vi "TDK-Lambda GEN LAN Series - GUI Demo.vi"() -> ()   [LabVIEW 2025]
doc: "This is a simple Graphical User Interface (GUI), for the TDK-Lambda Genesys DC Power Supplies using Ethernet (LAN) ports. \n\nIt has controls and indicators that automatically update in an endless polling loop. It also shows a pop-up form when errors are detected.\n\nControls: \n- Knobs to set voltage and current limits.\n- Buttons to set the output on or off, reset and quit.\n\nIndicators:\n- Shows the measured output voltage and current.\n- Shows the CV or CC regulation mode.\n- Shows when the output is turned off.\n- Shows fault shut down messages."
uses:
  <userlib>/TDK-Lambda GEN LAN Series/TDK-Lambda GEN LAN Series.lvlib
panel:
  in  "Revision":string="Rev 1.03"
  in  "RESET":bool
  out "Seqnc":string
  in  "VISA Name":refnum<visa-resource-name>="TCPIP0::0.0.0.0::inst0::INSTR" caption="IP Address"
  out "Irate Str":string caption="I Rate"
  out "Vrate Str":string caption="V Rate"
  out "Console":string
  in  "PC":dbl(knob) min=0.0 max=25.0 scale=0.0..25.0 scale format="%.1f"
  in  "IDecPt":enum16{"1", "10", "100", "1000"}(ring)=enum."100"
  in  "VDecPt":enum16{"1", "10", "100", "1000"}(ring)=enum."100"
  in  "QuitBtn":bool
  out "CcLed":bool=TRUE
  out "OUTled":bool=TRUE
  in  "OUT":bool
  out "IDisp":cluster{string[], bool, bool, bool, bool}={["0", "0", "0", "0", "0"], FALSE, FALSE, TRUE, FALSE}
  out "CvLed":bool=TRUE
  out "VDisp":cluster{string[], bool, bool, bool, bool}={["0", "0", "0", "0", "0"], FALSE, TRUE, FALSE, FALSE}
  in  "PV":dbl(knob) min=0.0 max=30.0 scale=0.0..30.0 scale format="%.1f"
  # "Command Logging"
  # "GENESYS Power Supply"
  # "DC VOLTS"
  # "DC AMPS"
  # "(c) 2019 TDK-Lambda.  ALL RIGHTS RESERVED."
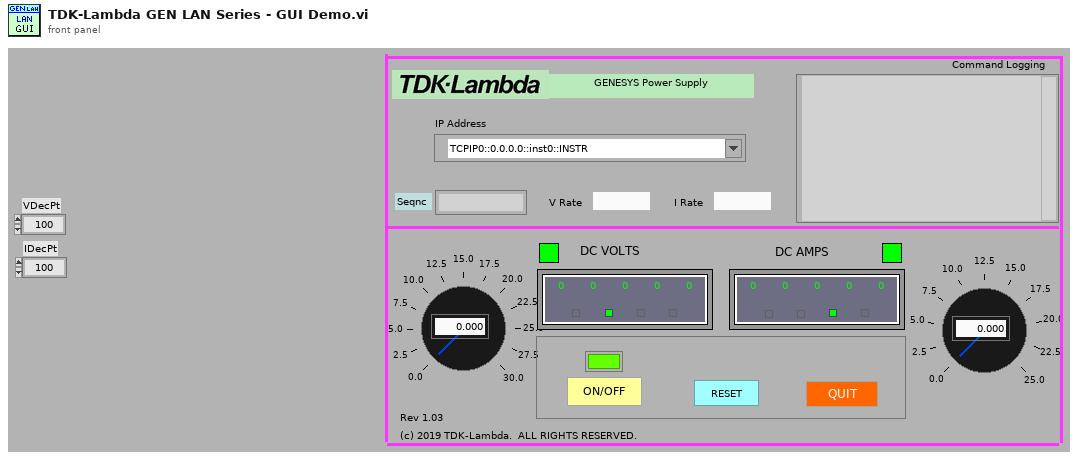
[diagram p1: front panel]
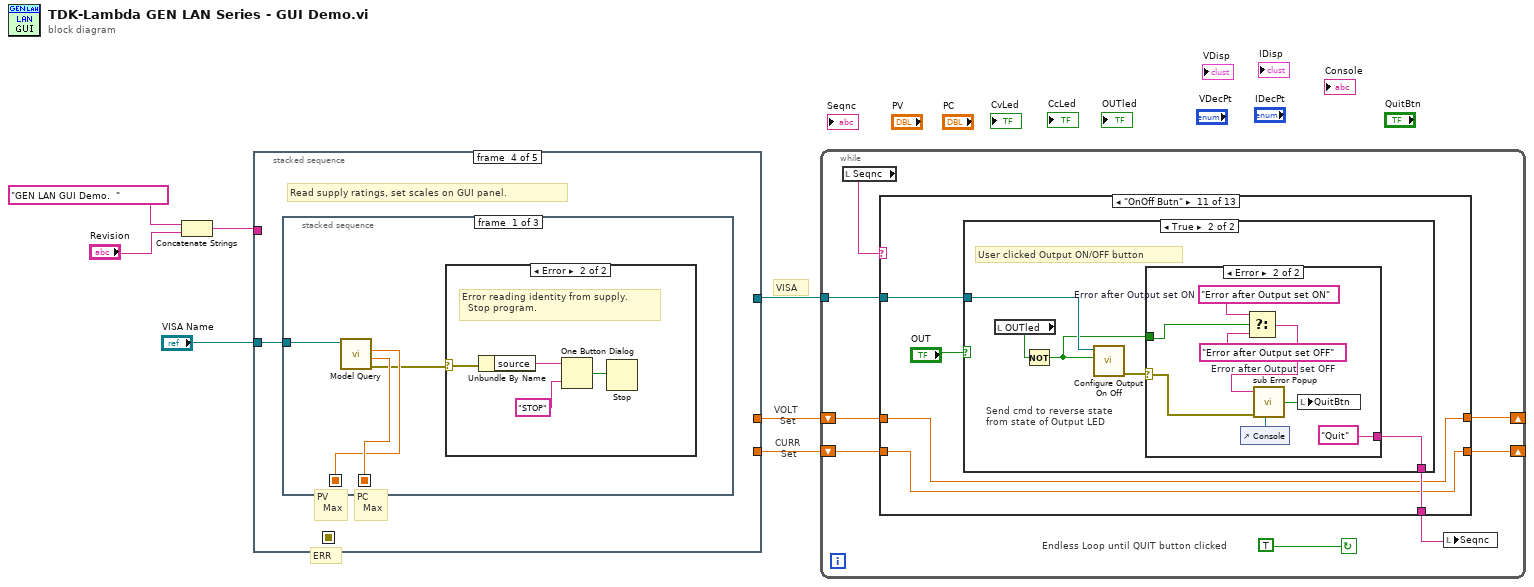
[diagram p0: block diagram]
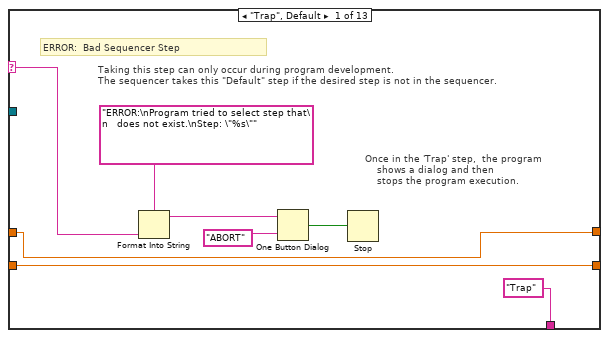
[diagram p2: hidden frame]
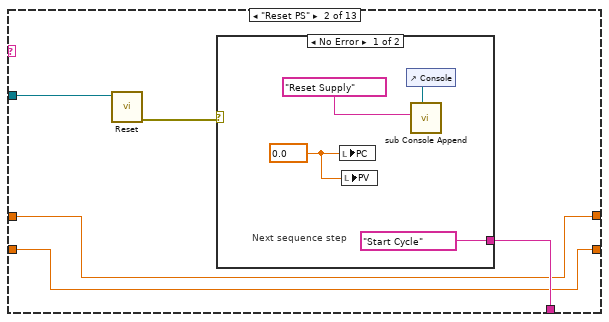
[diagram p3: hidden frame]
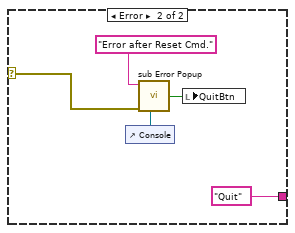
[diagram p4: hidden frame]
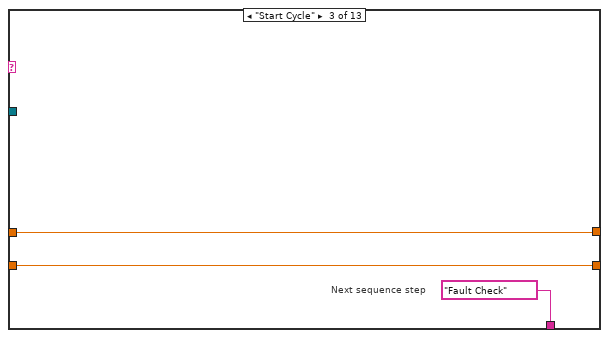
[diagram p5: hidden frame]
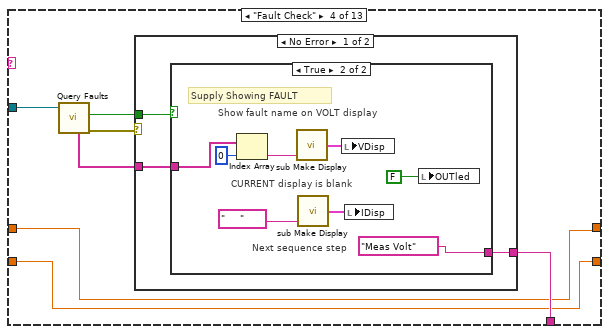
[diagram p6: hidden frame]
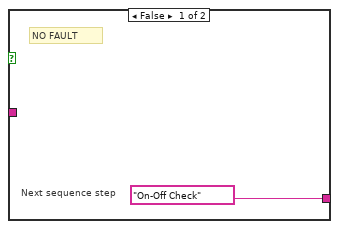
[diagram p7: hidden frame]
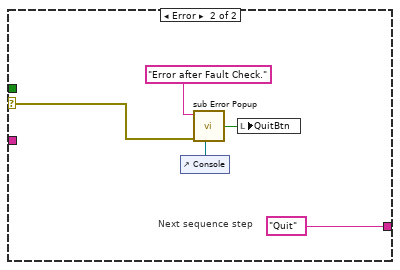
[diagram p8: hidden frame]
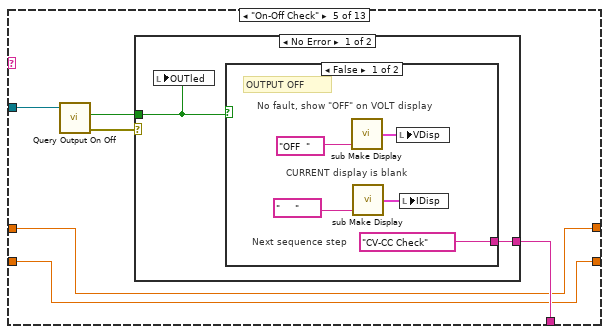
[diagram p9: hidden frame]
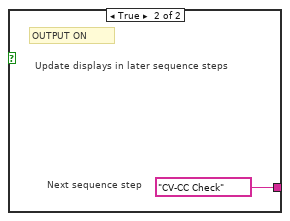
[diagram p10: hidden frame]
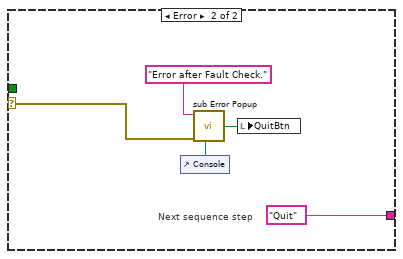
[diagram p11: hidden frame]
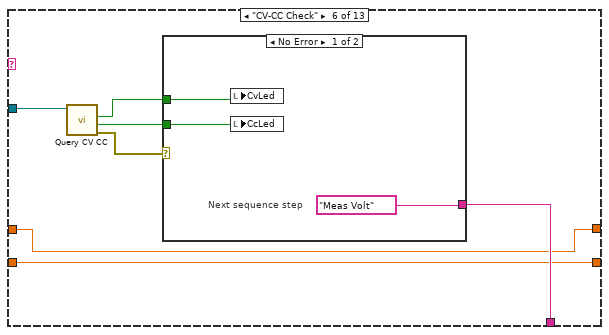
[diagram p12: hidden frame]
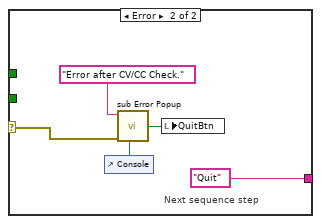
[diagram p13: hidden frame]
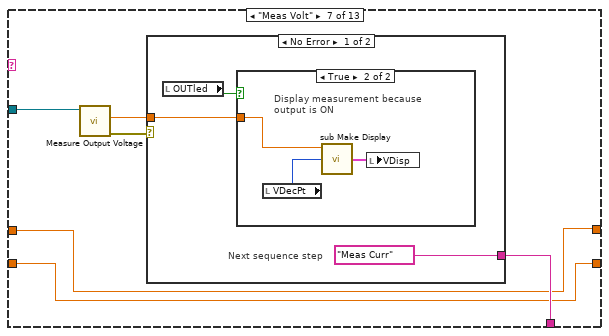
[diagram p14: hidden frame]
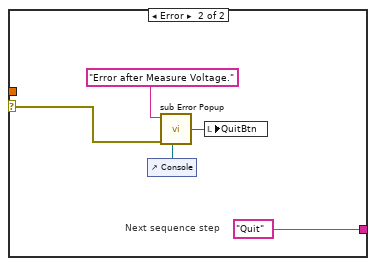
[diagram p16: hidden frame]
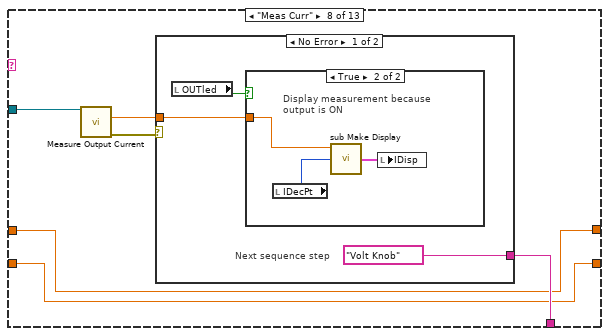
[diagram p17: hidden frame]
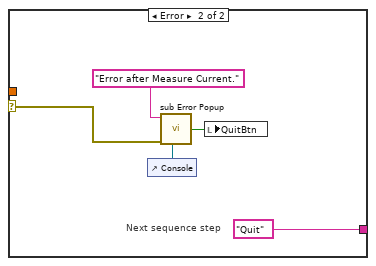
[diagram p19: hidden frame]
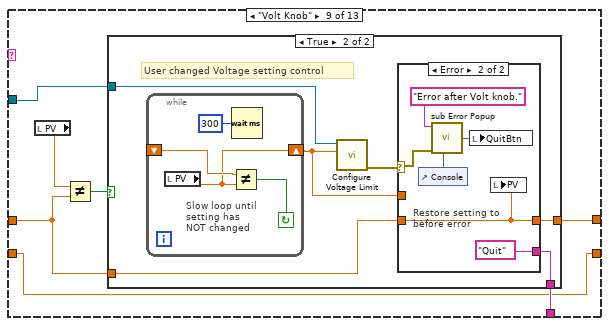
[diagram p20: hidden frame]
diagram:
  # "CURR \n  Set"
  # "VOLT \n  Set"
  # "VISA"
  # "ERR"
  n1 = Concatenate Strings("GEN LAN GUI Demo.  ", "Revision") -> (w1:string)
  n2 = stacked-sequence {
    seq-local: [_ w22 _ _ _] -> [_ _ w25 _ _]
    tunnel: [_ _ w26 _ _] -> w7
    tunnel: w1 -> [w12 _ _ _ _]
    tunnel: "VISA Name" -> [_ w20 w28 w35 _]
    tunnel: [_ _ _ _ 0.0 ("y")] -> w5
    tunnel: [_ _ _ _ 0.0 ("y")] -> w4
    frame #0 {
      w8 = 0.0 ("PV")
      w9 = FALSE ("AlmLed")
      w13 = "\r\n"
      w10 = ""
      n3 = Format Date/Time String() -> (date/time string=w14:string)  [unwired: 3 in]
      n4 = call "sub Make Display.vi"("String5"="     " ("String4")) -> ("Fmt Display"=w18:cluster{string[], bool, bool, bool, bool})  [unwired: 2 in]
      n5 = call "sub Make Display.vi"("String5"="     " ("String4")) -> ("Fmt Display"=w15:cluster{string[], bool, bool, bool, bool})  [unwired: 2 in]
      n6 = Concatenate Strings(w12, w13, w14, w13) -> (w11:string)
      n7 = local write "VDisp"(w15) -> ()
      n8 = local write "IDisp"(w18) -> ()
      n9 = local write "Console"(w11) -> ()
      n10 = local write "Vrate Str"(w10) -> ()
      n11 = local write "Irate Str"(w10) -> ()
      n12 = local write "OUTled"(w9) -> ()
      n13 = local write "QuitBtn"(w9) -> ()
      n14 = local write "CcLed"(w9) -> ()
      n15 = local write "CvLed"(w9) -> ()
      n16 = local write "PV"(w8) -> ()
      n17 = local write "PC"(w8) -> ()
    }
    frame #1 {
      # "Show LAN IP address on text Console"
      n18 = property class="TCP/IP Instr"(reference=w20) -> (error out=w22:errorcluster, "General Settings:Resource Name"=w23:string)  [unwired: 1 in, 1 out]
      n19 = Format Into String(format string="Open GEN LAN: %s", w23) -> (resulting string=w21:string)  [unwired: 2 in, 1 out]
      n20 = control-ref of="Console"() -> (w19:refnum<vi>)
      n21 = call "sub Console Append.vi"("Console Ref"=w19, "String"=w21) -> ()  [unwired: 4 in, 3 out]
    }
    frame #2 {
      # "Open LAN Port.  \n  If error, stop the program."
      n22 = call <userlib>:"Initialize.vi"("error in (no error)"=w25, "VISA name"=w28) -> ("error out"=w27:errorcluster, "VISA out"=w26:refnum<visa-resource-name>)  [unwired: 8 in]
      n23 = case shown="Error" w27 {
        selector: w27 -> [_ w32]
        frame No Error {
          # "LAN Port opened, \n  Power supply is talking."
        }
        frame Error {
          # "Cannot Open LAN Port,\n  or Cannot get response from supply.  \n  Stop the program."
          n24 = Unbundle By Name(w32) -> ("source"=w31:string)
          n25 = Concatenate Strings("Did you enter a valid VISA IP address or hostname before clicking the RUN button?\n", w31) -> (w30:string)
          n26 = One Button Dialog(message=w30, button name ("OK")="STOP") -> (true=w33:bool)
          n27 = Stop(stop? (T)=w33) -> ()
        }
      }
    }
    frame #3 {
      # "PC \n  Max"
      # "PV \n  Max"
      # "Read supply ratings, set scales on GUI panel."
      n28 = stacked-sequence {
        seq-local: [w37 _ _] -> [_ w48 w61]
        seq-local: [w38 _ _] -> [_ w47 w60]
        tunnel: w35 -> [w39 _ _]
        frame #0 {
          n29 = call <userlib>:"Model Query.vi"("VISA"=w39) -> ("error out"=w36:errorcluster, "Current Rating"=w38:dbl, "Voltage Rating"=w37:dbl)  [unwired: 5 in, 3 out]
          n30 = case shown="Error" w36 {
            selector: w36 -> [_ w40]
            frame No Error {
              # "Model ratings were\n     read from supply."
            }
            frame Error {
              # "Error reading identity from supply.\n  Stop program."
              n31 = Unbundle By Name(w40) -> ("source"=w41:string)
              n32 = One Button Dialog(message=w41, button name ("OK")="STOP") -> (true=w42:bool)
              n33 = Stop(stop? (T)=w42) -> ()
            }
          }
        }
        frame #1 {
          # "Find decimal points for 7-Seg displays"
          n34 = Format Into String(format string="%d" ("expression (\"\")"), w47) -> (resulting string=w44:string)  [unwired: 2 in, 1 out]
          n35 = Format Into String(format string="%d" ("expression (\"\")"), w48) -> (resulting string=w45:string)  [unwired: 2 in, 1 out]
          n36 = String Length(string=w44) -> (length=w57:i32)
          n37 = String Length(string=w45) -> (length=w58:i32)
          n38 = To Unsigned Word Integer(number=w57) -> (unsigned 16bit integer=w50:u16)
          n39 = To Unsigned Word Integer(number=w58) -> (unsigned 16bit integer=w54:u16)
          n40 = Subtract(x=u16 5 ("y"), y=w50) -> (x-y=w49:u16)
          n41 = Subtract(x=u16 5 ("y"), y=w54) -> (x-y=w46:u16)
          n42 = Decrement(x=w50) -> (x-1=w52:u16)
          n43 = Decrement(x=w54) -> (x-1=w53:u16)
          n44 = property on="PC" class="Knob (strict)"("Old Format & Precision:Old Precision"=w49) -> ()  [unwired: 2 in, 2 out]
          n45 = property on="PV" class="Knob (strict)"("Old Format & Precision:Old Precision"=w46) -> ()  [unwired: 2 in, 2 out]
          n46 = local write "VDecPt"(w53) -> ()
          n47 = property on="Property Node" class="DigNum (strict)"("Numeric Text.Display Format:Precision"=w49) -> ()  [unwired: 2 in, 2 out]
          n48 = property class="DigNum (strict)"("Numeric Text.Display Format:Precision"=w46) -> ()  [unwired: 2 in, 2 out]
          n49 = local write "IDecPt"(w52) -> ()
        }
        frame #2 {
          # "Max Curr =Rated Curr"
          # "Max Volt = Rated Volt"
          # "Set data range of knobs"
          n50 = Format Into String(format string="%.1f" ("expression (\"\")"), w61) -> (resulting string=→"Vrate Str":string)  [unwired: 2 in, 1 out]
          n51 = Format Into String(format string="%.1f" ("expression (\"\")"), w60) -> (resulting string=→"Irate Str":string)  [unwired: 2 in, 1 out]
          n52 = property on="PV" class="Knob (strict)"("Data Entry Limits:Maximum"=w61, "Scale.Range:Maximum"=w61, "Scale.Range:Minimum"=0.0) -> ()  [unwired: 2 in, 2 out]
          n53 = property on="PC" class="Knob (strict)"("Data Entry Limits:Maximum"=w60, "Scale.Range:Maximum"=w60, "Scale.Range:Minimum"=0.0) -> ()  [unwired: 2 in, 2 out]
        }
      }
    }
    frame #4 {
      # "First step is to reset the supply"
      n54 = local write "Seqnc"("Reset PS") -> ()
    }
  }
  n55 = while {
    tunnel: w7 -> [w77]
    shift-right: [w74] -> _
    shift-left: w5 -> [w75]
    shift-right: [w73] -> _
    shift-left: w4 -> [w72]
    stop <- TRUE continue-if-true
    # "Endless Loop until QUIT button clicked"
    n56 = local read "Seqnc"() -> (w78:string)
    n57 = case shown="\"OnOff Butn\"" w78 {
      selector: w78 -> [w83 _ _ _ _ _ _ _ _ _ _ _ _]
      tunnel: w77 -> [_ w91 _ w110 w133 w153 w167 w184 w199 w231 w259 _ w291]
      tunnel: ["Trap" w89 "Fault Check" w106 w130 w149 w164 w181 w197 w230 w258 w283 w290] -> w76
      tunnel: w75 -> [w81 w88 w102 w105 w129 w148 w163 w180 w198 w226 w257 w282 w288]
      tunnel: [w81 w88 w102 w105 w129 w148 w163 w180 w201 w226 w257 w282 w288] -> w74
      tunnel: [w80 w87 w101 w104 w128 w147 w162 w179 w196 w228 w256 w281 w287] -> w73
      tunnel: w72 -> [w80 w87 w101 w104 w128 w147 w162 w179 w196 w227 w256 w281 w287]
      frame "Trap", Default {
        # "Once in the 'Trap' step,  the program \n    shows a dialog and then \n    stops the program execution."
        # "Taking this step can only occur during program development.\nThe sequencer takes this \"Default\" step if the desired step is not in the sequencer."
        # "ERROR:  Bad Sequencer Step"
        n58 = Format Into String(format string="ERROR:\nProgram tried to select step that\n   does not exist.\nStep: \"%s\"", w83) -> (resulting string=w85:string)  [unwired: 2 in, 1 out]
        n59 = One Button Dialog(message=w85, button name ("OK")="ABORT") -> (true=w79:bool)
        n60 = Stop(stop? (T)=w79) -> ()
      }
      frame "Reset PS" {
        n61 = call <userlib>:"Reset.vi"("VISA"=w91) -> ("error out"=w90:errorcluster)  [unwired: 9 in, 1 out]
        n62 = case shown="No Error" w90 {
          selector: w90 -> [_ w97]
          tunnel: ["Start Cycle" "Quit"] -> w89
          frame No Error {
            w93 = 0.0 ("y")
            # "Next sequence step"
            n63 = local write "PC"(w93) -> ()
            n64 = local write "PV"(w93) -> ()
            n65 = control-ref of="Console"() -> (w95:refnum<vi>)
            n66 = call "sub Console Append.vi"("Console Ref"=w95, "String"="Reset Supply") -> ()  [unwired: 4 in, 3 out]
          }
          frame Error {
            n67 = control-ref of="Console"() -> (w100:refnum<vi>)
            n68 = call "sub Error Popup.vi"("Error Message"="Error after Reset Cmd." ("My Mesg"), "error in"=w97, "Console Ref"=w100) -> ("Quit Out"=w99:bool)  [unwired: 2 in, 2 out]
            n69 = local write "QuitBtn"(w99) -> ()
          }
        }
      }
      frame "Start Cycle" {
        # "Next sequence step"
      }
      frame "Fault Check" {
        n70 = call <userlib>:"Query Faults.vi"("VISA"=w110) -> ("error out"=w109:errorcluster, "Fault?"=w108:bool, "Descriptions"=w107:string[])  [unwired: 6 in, 2 out]
        n71 = case shown="No Error" w109 {
          selector: w109 -> [_ w124]
          tunnel: [w113 "Quit"] -> w106
          tunnel: w108 -> [w112 _]
          tunnel: w107 -> [w111 _]
          frame No Error {
            n72 = case shown="True" w112 {
              tunnel: ["On-Off Check" "Meas Volt"] -> w113
              tunnel: w111 -> [_ w121]
              frame False {
                # "Next sequence step"
                # "NO FAULT"
              }
              frame True {
                # "Next sequence step"
                # "CURRENT display is blank"
                # "Show fault name on VOLT display"
                # "Supply Showing FAULT"
                n73 = Index Array(array=w121, index=0) -> (element=w119:string)
                n74 = call "sub Make Display.vi"("String5"=w119) -> ("Fmt Display"=w122:cluster{string[], bool, bool, bool, bool})  [unwired: 2 in]
                n75 = call "sub Make Display.vi"("String5"="     ") -> ("Fmt Display"=w118:cluster{string[], bool, bool, bool, bool})  [unwired: 2 in]
                n76 = local write "VDisp"(w122) -> ()
                n77 = local write "IDisp"(w118) -> ()
                n78 = local write "OUTled"(FALSE ("OUTled")) -> ()
              }
            }
          }
          frame Error {
            # "Next sequence step"
            n79 = control-ref of="Console"() -> (w127:refnum<vi>)
            n80 = call "sub Error Popup.vi"("Error Message"="Error after Fault Check." ("My Mesg"), "error in"=w124, "Console Ref"=w127) -> ("Quit Out"=w126:bool)  [unwired: 2 in, 2 out]
            n81 = local write "QuitBtn"(w126) -> ()
          }
        }
      }
      frame "On-Off Check" {
        n82 = call <userlib>:"Query Output On Off.vi"("VISA"=w133) -> ("error out"=w131:errorcluster, "Output ON"=w132:bool)  [unwired: 8 in, 1 out]
        n83 = case shown="No Error" w131 {
          selector: w131 -> [_ w143]
          tunnel: [w135 "Quit"] -> w130
          tunnel: w132 -> [w134 _]
          frame No Error {
            n84 = local write "OUTled"(w134) -> ()
            n85 = case shown="False" w134 {
              tunnel: ["CV-CC Check" "CV-CC Check"] -> w135
              frame False {
                # "Next sequence step"
                # "CURRENT display is blank"
                # "No fault, show \"OFF\" on VOLT display"
                # "OUTPUT OFF"
                n86 = call "sub Make Display.vi"("String5"="OFF  ") -> ("Fmt Display"=w139:cluster{string[], bool, bool, bool, bool})  [unwired: 2 in]
                n87 = call "sub Make Display.vi"("String5"="     ") -> ("Fmt Display"=w138:cluster{string[], bool, bool, bool, bool})  [unwired: 2 in]
                n88 = local write "VDisp"(w139) -> ()
                n89 = local write "IDisp"(w138) -> ()
              }
              frame True {
                # "Next sequence step"
                # "Update displays in later sequence steps"
                # "OUTPUT ON"
              }
            }
          }
          frame Error {
            # "Next sequence step"
            n90 = control-ref of="Console"() -> (w146:refnum<vi>)
            n91 = call "sub Error Popup.vi"("Error Message"="Error after Fault Check." ("My Mesg"), "error in"=w143, "Console Ref"=w146) -> ("Quit Out"=w145:bool)  [unwired: 2 in, 2 out]
            n92 = local write "QuitBtn"(w145) -> ()
          }
        }
      }
      frame "CV-CC Check" {
        n93 = call <userlib>:"Query CV CC.vi"("VISA"=w153) -> ("error out"=w152:errorcluster, "CC"=w150:bool, "CV"=w151:bool)  [unwired: 5 in, 3 out]
        n94 = case shown="No Error" w152 {
          selector: w152 -> [_ w158]
          tunnel: ["Meas Volt" "Quit"] -> w149
          tunnel: w151 -> [w156 _]
          tunnel: w150 -> [w155 _]
          frame No Error {
            # "Next sequence step"
            n95 = local write "CvLed"(w156) -> ()
            n96 = local write "CcLed"(w155) -> ()
          }
          frame Error {
            # "Next sequence step"
            n97 = control-ref of="Console"() -> (w161:refnum<vi>)
            n98 = call "sub Error Popup.vi"("Error Message"="Error after CV/CC Check." ("My Mesg"), "error in"=w158, "Console Ref"=w161) -> ("Quit Out"=w160:bool)  [unwired: 2 in, 2 out]
            n99 = local write "QuitBtn"(w160) -> ()
          }
        }
      }
      frame "Meas Volt" {
        n100 = call <userlib>:"Measure Output Voltage.vi"("VISA"=w167) -> ("error out"=w166:errorcluster, "Output Voltage"=w165:dbl)  [unwired: 8 in, 1 out]
        n101 = case shown="No Error" w166 {
          selector: w166 -> [_ w175]
          tunnel: ["Meas Curr" "Quit"] -> w164
          tunnel: w165 -> [w169 _]
          frame No Error {
            # "Next sequence step"
            n102 = local read "OUTled"() -> (w168:bool)
            n103 = case shown="True" w168 {
              tunnel: w169 -> [_ w171]
              frame False {
                # "Output is OFF.\nDo not write measurement \n   to voltage display"
              }
              frame True {
                # "Display measurement because\noutput is ON"
                n104 = local read "VDecPt"() -> (w172:enum16{"1", "10", "100", "1000"})
                n105 = call "sub Make Display.vi"("Decimal Point"=w172, "Number Value"=w171) -> ("Fmt Display"=w173:cluster{string[], bool, bool, bool, bool})  [unwired: 1 in]
                n106 = local write "VDisp"(w173) -> ()
              }
            }
          }
          frame Error {
            # "Next sequence step"
            n107 = control-ref of="Console"() -> (w178:refnum<vi>)
            n108 = call "sub Error Popup.vi"("Error Message"="Error after Measure Voltage." ("My Mesg"), "error in"=w175, "Console Ref"=w178) -> ("Quit Out"=w177:bool)  [unwired: 2 in, 2 out]
            n109 = local write "QuitBtn"(w177) -> ()
          }
        }
      }
      frame "Meas Curr" {
        n110 = call <userlib>:"Measure Output Current.vi"("VISA"=w184) -> ("error out"=w183:errorcluster, "Output Current"=w182:dbl)  [unwired: 8 in, 1 out]
        n111 = case shown="No Error" w183 {
          selector: w183 -> [_ w193]
          tunnel: ["Volt Knob" "Quit"] -> w181
          tunnel: w182 -> [w186 _]
          frame No Error {
            # "Next sequence step"
            n112 = local read "OUTled"() -> (w185:bool)
            n113 = case shown="True" w185 {
              tunnel: w186 -> [_ w189]
              frame False {
                # "Output is OFF.\nDo not write measurement \n   to current display"
              }
              frame True {
                # "Display measurement because\noutput is ON"
                n114 = local read "IDecPt"() -> (w188:enum16{"1", "10", "100", "1000"})
                n115 = call "sub Make Display.vi"("Decimal Point"=w188, "Number Value"=w189) -> ("Fmt Display"=w190:cluster{string[], bool, bool, bool, bool})  [unwired: 1 in]
                n116 = local write "IDisp"(w190) -> ()
              }
            }
          }
          frame Error {
            # "Next sequence step"
            n117 = control-ref of="Console"() -> (w195:refnum<vi>)
            n118 = call "sub Error Popup.vi"("Error Message"="Error after Measure Current." ("My Mesg"), "error in"=w193, "Console Ref"=w195) -> ("Quit Out"=w194:bool)  [unwired: 2 in, 2 out]
            n119 = local write "QuitBtn"(w194) -> ()
          }
        }
      }
      frame "Volt Knob" {
        n120 = local read "PV"() -> (w200:dbl)
        n121 = Not Equal?(x=w200, y=w198) -> (x != y?=w202:bool)
        n122 = case shown="True" w202 {
          tunnel: [w203 w207] -> w201
          tunnel: w199 -> [_ w210]
          tunnel: w198 -> [w203 w208]
          tunnel: ["Curr Knob" w205] -> w197
          frame False {
            # "Next sequence step"
            # "Window voltage control not changed,  do not sent programming cmd"
          }
          frame True {
            # "User changed Voltage setting control"
            n123 = while {
              shift-right: [w224] -> w206
              shift-left: _ -> [w225]
              stop <- w223 continue-if-true
              # "Slow loop until \nsetting has \nNOT changed"
              n124 = local read "PV"() -> (w224:dbl)
              n125 = Not Equal?(x=w225, y=w224) -> (x != y?=w223:bool)
              n126 = Wait (ms)(milliseconds to wait=u32 300) -> ()  [unwired: 1 out]
            }
            n127 = call <userlib>:"Configure Voltage Limit.vi"("Voltage Limit"=w206, "VISA"=w210) -> ("error out"=w209:errorcluster)  [unwired: 8 in, 1 out]
            n128 = case shown="Error" w209 {
              selector: w209 -> [_ w218]
              tunnel: w208 -> [_ w216]
              tunnel: [w213 w216] -> w207
              tunnel: w206 -> [w213 _]
              tunnel: ["Curr Knob" "Quit"] -> w205
              frame No Error {
                # "Use System\nDecimal Pt."
                n129 = Format Into String(format string="%.;PV %0.4f", w213) -> (resulting string=w212:string)  [unwired: 2 in, 1 out]
                n130 = control-ref of="Console"() -> (w215:refnum<vi>)
                n131 = call "sub Console Append.vi"("Console Ref"=w215, "String"=w212) -> ()  [unwired: 4 in, 3 out]
              }
              frame Error {
                # "Restore setting to\nbefore error"
                n132 = control-ref of="Console"() -> (w221:refnum<vi>)
                n133 = call "sub Error Popup.vi"("Error Message"="Error after Volt knob." ("My Mesg"), "error in"=w218, "Console Ref"=w221) -> ("Quit Out"=w220:bool)  [unwired: 2 in, 2 out]
                n134 = local write "QuitBtn"(w220) -> ()
                n135 = local write "PV"(w216) -> ()
              }
            }
          }
        }
      }
      frame "Curr Knob" {
        n136 = local read "PC"() -> (w229:dbl)
        n137 = Not Equal?(x=w229, y=w227) -> (x != y?=w232:bool)
        n138 = case shown="True" w232 {
          tunnel: w227 -> [w234 _]
          tunnel: [w234 w239] -> w228
          tunnel: w231 -> [_ w236]
          tunnel: w227 -> [_ w240]
          tunnel: ["OnOff Butn" w238] -> w230
          frame False {
            # "Next sequence step"
            # "Window voltage control not changed,  do not sent programming cmd"
          }
          frame True {
            # "User changed Current setting control"
            n139 = while {
              shift-right: [w254] -> w237
              shift-left: _ -> [w255]
              stop <- w253 continue-if-true
              # "Slow loop until \nsetting has \nNOT changed"
              n140 = local read "PC"() -> (w254:dbl)
              n141 = Not Equal?(x=w255, y=w254) -> (x != y?=w253:bool)
              n142 = Wait (ms)(milliseconds to wait=u32 300) -> ()  [unwired: 1 out]
            }
            n143 = call <userlib>:"Configure Current Limit.vi"("Current Limit"=w237, "VISA"=w236) -> ("error out"=w235:errorcluster)  [unwired: 8 in, 1 out]
            n144 = case shown="Error" w235 {
              selector: w235 -> [_ w248]
              tunnel: w240 -> [_ w246]
              tunnel: [w243 w246] -> w239
              tunnel: w237 -> [w243 _]
              tunnel: ["OnOff Butn" "Quit"] -> w238
              frame No Error {
                # "Use System\nDecimal Pt."
                n145 = Format Into String(format string="%.;PC %0.4f", w243) -> (resulting string=w242:string)  [unwired: 2 in, 1 out]
                n146 = control-ref of="Console"() -> (w245:refnum<vi>)
                n147 = call "sub Console Append.vi"("Console Ref"=w245, "String"=w242) -> ()  [unwired: 4 in, 3 out]
              }
              frame Error {
                # "Restore setting to\nbefore error"
                n148 = control-ref of="Console"() -> (w251:refnum<vi>)
                n149 = call "sub Error Popup.vi"("Error Message"="Error after Volt knob." ("My Mesg"), "error in"=w248, "Console Ref"=w251) -> ("Quit Out"=w250:bool)  [unwired: 2 in, 2 out]
                n150 = local write "QuitBtn"(w250) -> ()
                n151 = local write "PC"(w246) -> ()
              }
            }
          }
        }
      }
      frame "OnOff Butn" {
        n152 = case shown="True" "OUT" {
          tunnel: w259 -> [_ w265]
          tunnel: ["Reset Butn" w262] -> w258
          frame False {
            # "Output ON/OFF button not clicked"
          }
          frame True {
            # "Send cmd to reverse state\nfrom state of Output LED"
            # "User clicked Output ON/OFF button"
            n153 = local read "OUTled"() -> (w266:bool)
            n154 = Not(x=w266) -> (.not. x?=w263:bool)
            n155 = call <userlib>:"Configure Output On Off.vi"("Output ON"=w263, "VISA"=w265) -> ("error out"=w264:errorcluster)  [unwired: 8 in, 1 out]
            n156 = case shown="Error" w264 {
              selector: w264 -> [_ w278]
              tunnel: ["Reset Butn" "Quit"] -> w262
              tunnel: w263 -> [w270 w274]
              frame No Error {
                # "Next sequence step"
                n157 = Select(t="Output set ON", s=w270, f="Output set OFF") -> (s? t:f=w267:string)
                n158 = control-ref of="Console"() -> (w272:refnum<vi>)
                n159 = call "sub Console Append.vi"("Console Ref"=w272, "String"=w267) -> ()  [unwired: 4 in, 3 out]
              }
              frame Error {
                w275 = "Error after Output set OFF"  # Error after Output set OFF
                w276 = "Error after Output set ON"  # Error after Output set ON
                n160 = control-ref of="Console"() -> (w280:refnum<vi>)
                n161 = Select(t=w276, s=w274, f=w275) -> (s? t:f=w273:string)
                n162 = call "sub Error Popup.vi"("Error Message"=w273, "error in"=w278, "Console Ref"=w280) -> ("Quit Out"=w279:bool)  [unwired: 2 in, 2 out]
                n163 = local write "QuitBtn"(w279) -> ()
              }
            }
          }
        }
      }
      frame "Reset Butn" {
        n164 = Select(t="Reset PS", s="RESET", f="Quit") -> (s? t:f=w283:string)
      }
      frame "Quit" {
        n165 = local read "QuitBtn"() -> (w292:bool)
        n166 = case shown="True" w292 {
          tunnel: w291 -> [_ w297]
          tunnel: ["Start Cycle" "Quit"] -> w290
          tunnel: [FALSE TRUE] -> w289
          frame False {
          }
          frame True {
            # "User clicked Quit button,  \n    or error pop-up caused it to be set"
            n167 = call <userlib>:"Close.vi"("VISA name"=w297) -> ()  [unwired: 10 in, 1 out]
          }
        }
        n168 = Stop(stop? (T)=w289) -> ()
      }
    }
    n169 = local write "Seqnc"(w76) -> ()
  }
